vi "SetConfig.vi"(8 "error in (no error)":errorcluster, 10 "Variant":variant, 11 "ArbitraryFunction in":refnum<class "ArbitraryFunction.lvclass">) -> (0 "error out":errorcluster, 3 "ArbitraryFunction out":refnum<class "ArbitraryFunction.lvclass">)   [LabVIEW 2018, in "Functions.lvlib" / "ArbitraryFunction.lvclass"]
uses:
  ArbitraryFunction.lvclass
  TypeDefs/ArbCfg.ctl
  TypeDefs/Arbitrary.ctl
  ArbitraryFunction.lvclass/ArbitraryFunction.ctl
  Accessors/Write Count.vi
  Accessors/Write Arbs.vi
  Accessors/Write SampleRate.vi
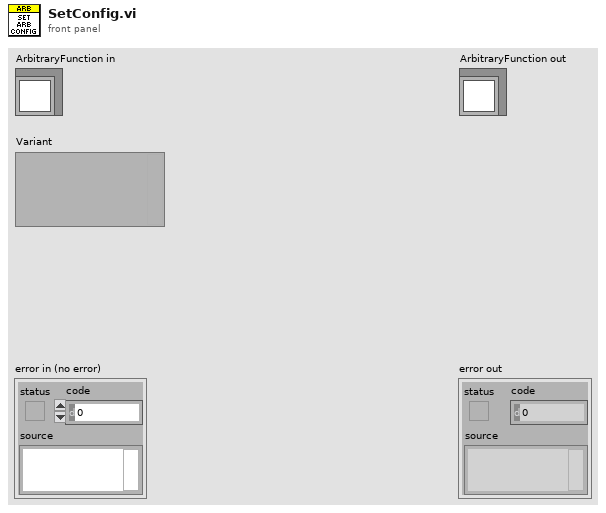
[diagram p1: front panel]
types:
  T1 = typedef "Functions.lvlib/ArbitraryFunction.lvclass/ArbCfg.ctl" = cluster{"SampleRate":dbl, "Count":u16, "Arbs":T2[]}
  T2 = typedef "Functions.lvlib/ArbitraryFunction.lvclass/Arbitrary.ctl" = cluster{"Handle":string, "Size":i32, "Gain":dbl, "Offset":dbl, "Waveform":waveform(dbl)}
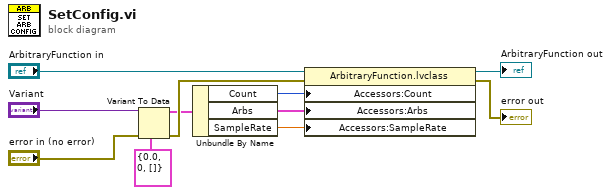
[diagram p0: block diagram]
diagram:
  n1 = Variant To Data(error in="error in (no error)", type=T1 {"SampleRate"=0.0, "Count"=0, "Arbs"=[]} ("ArbCfg"), Variant="Variant") -> (data=w4:T1, error out=w8:errorcluster)
  n2 = Unbundle By Name(w4) -> ("Count"=w3:u16, "Arbs"=w2:T2[], "SampleRate"=w1:dbl)
  n3 = property class="ArbitraryFunction.lvclass"(reference="ArbitraryFunction in", error in=w8, "Accessors:Count"=w3, "Accessors:Arbs"=w2, "Accessors:SampleRate"=w1) -> (reference out=→"ArbitraryFunction out":refnum<class "ArbitraryFunction.lvclass">, error out=→"error out":errorcluster)
